vi "Write_Results_file.vi"(0 "Experiment start time":dbl, 1 "Experiment End time":dbl, 3 "Setup filename":string) -> ()   [LabVIEW 2016]
uses:
  Globals/Meas_global.vi
  Globals/Dynamic_call_global.ph.vi
  Controls/Post_Process.ctl
  Globals/Trav_pos_global.vi
  Controls/Inst_type.ctl
panel:
  out "x-y":u32
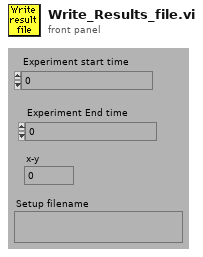
[diagram p1: front panel]
types:
  T1 = typedef "Post_Process.ctl" = enum16{"Take New Data", "Post Process Raw Data File"}
  T2 = enum16{"Save no data", "Save data in new files", "Save data in existing files"}
  T3 = typedef "Inst_type.ctl" = enum16{"Propeller anemometer", "Raw voltage", "Pressure Transducer", "Pitot-static tube", "Preston tube", "Hot wire", "Cross wire 1", "Cross wire 2", "Generic Linear", "Generic Polynomial", "Generic BackPoly", "Fast FID", "Thermocouple", "Cold wire", "Pulsed Wire", "LDA Vel", "LDA Tran time", "LDA Arr time", "Microphone"}
  T4 = typedef "Analysis_info_cluster.ctl" = cluster{"Colour":u32, "Inst type":T3, "Inst name":string, "Symbol":string, "Code name":string, "Extra Info":string, "Inst Array":T5, "Extra Titles":string[], "Extra Values":string[], "U":dbl, "u^2":dbl, "u^3":dbl, "u^4":dbl, "Skew_u":dbl, "Kurt_u":dbl, "Sd Error in Mean":dbl, "% u'/U":dbl, "X":dbl, "Y":dbl, "Z":dbl, "Timescale integral Estimate":dbl, "Sd Error in Variance":dbl, "Calib File":path, "Calib Constants":dbl[], "Output Position":bool, "Full Stats":bool, "Av Sampling Rate":dbl, "Av No of Samples":dbl, "Total Meas Time (s)":dbl, "ADAM Ch Name":string, "Max value":dbl, "Min value":dbl}
  T5 = typedef "Instrument_Array.ctl" = enum16{"PWA", "LDA", "Analogue"}
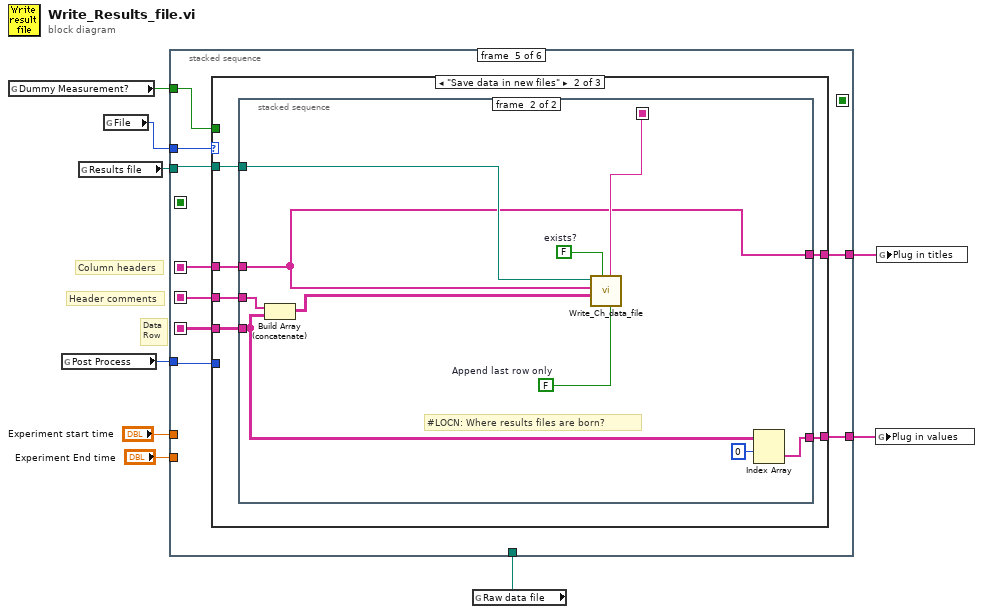
[diagram p0: block diagram]
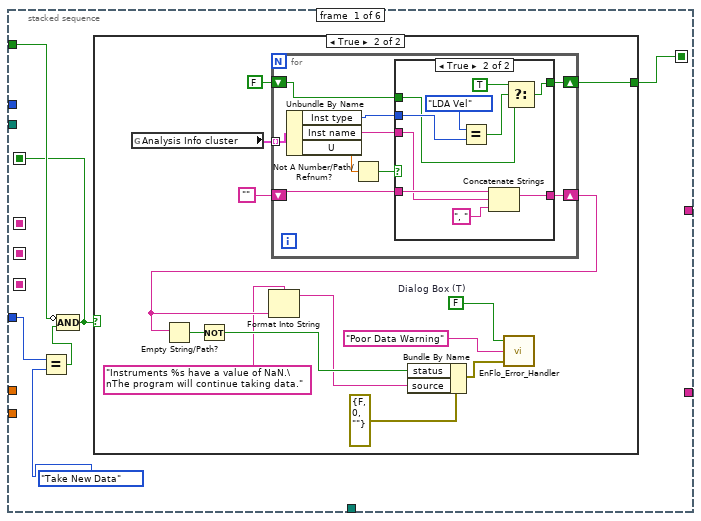
[diagram p2: hidden frame]
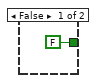
[diagram p3: hidden frame]
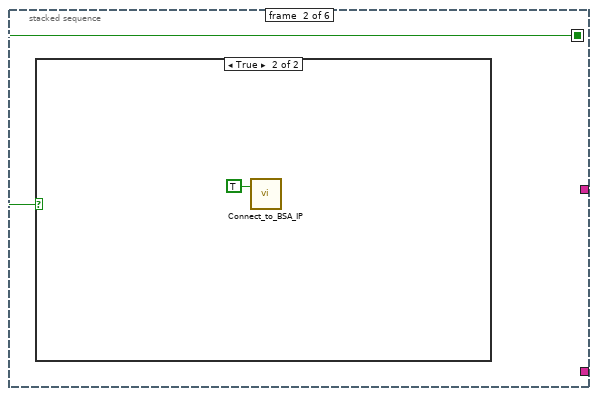
[diagram p5: hidden frame]
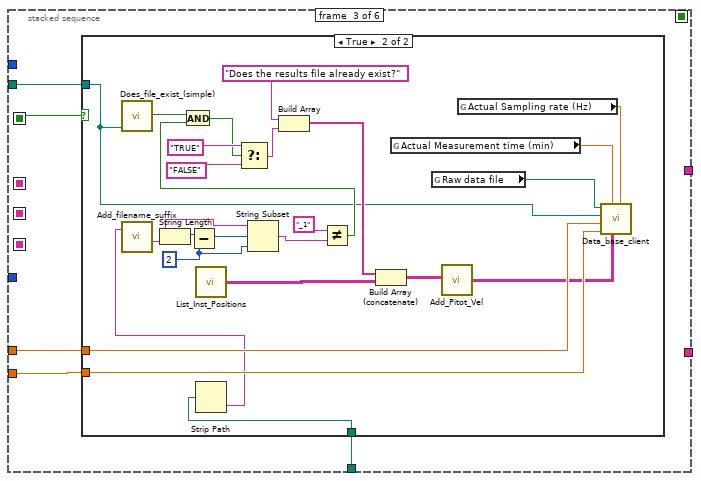
[diagram p7: hidden frame]
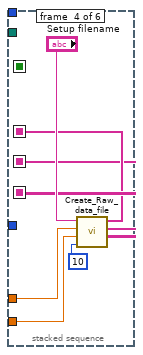
[diagram p9: hidden frame]
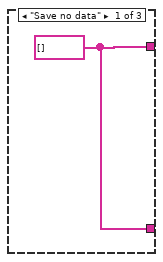
[diagram p10: hidden frame]
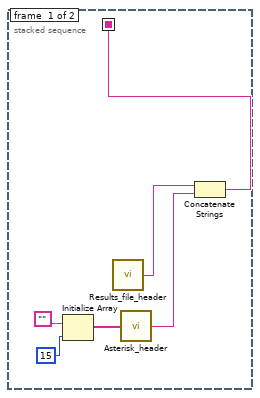
[diagram p11: hidden frame]
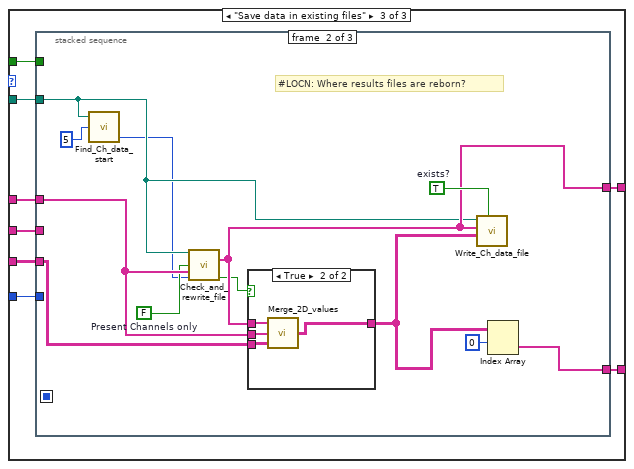
[diagram p12: hidden frame]
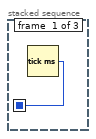
[diagram p13: hidden frame]
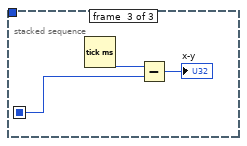
[diagram p15: hidden frame]
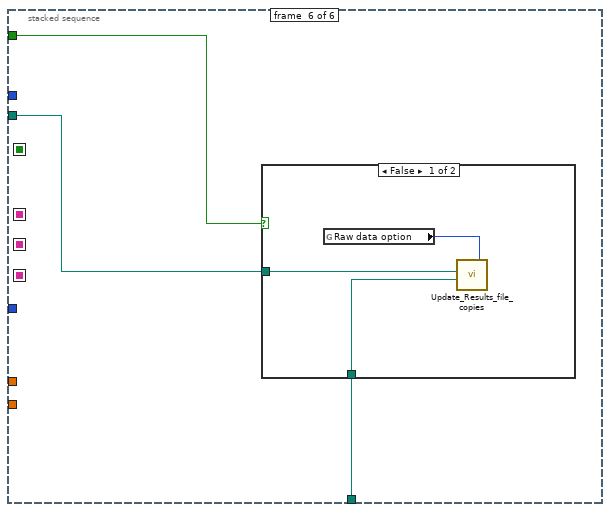
[diagram p16: hidden frame]
diagram:
  # "Data\nRow"
  # "Header comments"
  # "Column headers"
  n1 = global read "Trav_pos_global.vi" "Dummy Measurement?"() -> (w1:bool)
  n2 = global read "Meas_global.vi" "Post Process"() -> (w5:T1)
  n3 = global read "Meas_global.vi" "Results file"() -> (w2:path)
  n4 = global read "Meas_global.vi" "File"() -> (w9:T2)
  n5 = global read "Meas_global.vi" "Raw data file"() -> (w8:path)
  n6 = stacked-sequence {
    seq-local: [_ _ _ w84 _ _] -> [_ _ _ _ w97 _]
    seq-local: [_ _ _ w85 _ _] -> [_ _ _ _ w96 _]
    seq-local: [_ _ _ w83 _ _] -> [_ _ _ _ w95 _]
    seq-local: [w11 _ _ _ _ _] -> [_ _ w54 _ _ _]
    seq-local: [w10 _ _ _ _ _] -> [_ w51 _ _ _ _]
    tunnel: w9 -> [_ _ _ _ w98 _]
    tunnel: w8 -> [_ _ w53 _ _ w153]
    tunnel: "Experiment start time" -> [_ _ w57 w89 _ _]
    tunnel: "Experiment End time" -> [_ _ w56 w88 _ _]
    tunnel: w5 -> [w14 _ _ _ w94 _]
    tunnel: [_ _ _ _ w93 _] -> w4
    tunnel: [_ _ _ _ w92 _] -> w3
    tunnel: w2 -> [_ _ w55 _ w91 w152]
    tunnel: w1 -> [w12 _ _ _ w90 w151]
    frame #0 {
      n7 = Equal?(x=w14, y=Post_Process."Take New Data" ("Post Process")) -> (x = y?=w13:bool)
      n8 = Compound Arithmetic op=AND(invert w12, w13) -> (w11:bool)
      n9 = case shown="True" w11 {
        tunnel: [FALSE w17] -> w10
        frame False {
        }
        frame True {
          w26 = FALSE  # Dialog Box (T)
          n10 = global read "Meas_global.vi" "Analysis Info cluster"() -> (w29:T4[])
          n11 = for {
            tunnel: w29 -> [w38] mode=indexing
            shift-right: [w33] -> w21
            shift-left: "" -> [w35]
            shift-right: [w31] -> w17
            shift-left: FALSE -> [w30]
            n12 = Unbundle By Name(w38) -> ("Inst type"=w32:T3, "Inst name"=w34:string, "U"=w37:dbl)
            n13 = Not A Number/Path/Refnum?(number/path/refnum=w37) -> (NaN/Path/Refnum?=w36:bool)
            n14 = case shown="True" w36 {
              tunnel: w35 -> [w40 w50]
              tunnel: w34 -> [_ w49]
              tunnel: [w40 w47] -> w33
              tunnel: w32 -> [_ w45]
              tunnel: [w39 w42] -> w31
              tunnel: w30 -> [w39 w41]
              frame False {
              }
              frame True {
                n15 = Equal?(x=Inst_type."LDA Vel" ("Inst type"), y=w45) -> (x = y?=w44:bool)
                n16 = Concatenate Strings(w50, w49, ", " ("Substring")) -> (w47:string)
                n17 = Select(t=TRUE, s=w44, f=w41) -> (s? t:f=w42:bool)
              }
            }
          }
          n18 = Empty String/Path?(string/path=w21) -> (empty?=w23:bool)
          n19 = Not(x=w23) -> (.not. x?=w22:bool)
          n20 = Format Into String(format string="Instruments %s have a value of NaN.\nThe program will continue taking data." ("Format String"), w21) -> (resulting string=w19:string)  [unwired: 2 in, 1 out]
          n21 = Bundle By Name(cluster=errorcluster {"status"=FALSE, "code"=0, "source"=""} ("error in (no error)"), "status"=w22, "source"=w19) -> (w24:errorcluster)
          n22 = call "EnFlo_Error_Handler.vi"("error in (no error)"=w24, "Error Type"="Poor Data Warning", "Dialog Box (T)"=w26) -> ()  [unwired: 3 out]
        }
      }
    }
    frame #1 {
      n23 = case shown="True" w51 {
        frame False {
        }
        frame True {
          n24 = call "Connect_to_BSA_IP.vi"("Force Reconnect"=TRUE) -> ()  [unwired: 1 in, 2 out]
        }
      }
    }
    frame #2 {
      n25 = case shown="True" w54 {
        tunnel: w57 -> [_ w80]
        tunnel: w56 -> [_ w79]
        tunnel: w55 -> [_ w59]
        tunnel: w53 -> [_ w70]
        frame False {
        }
        frame True {
          w65 = 2 ("y")
          n26 = call "Does_file_exist_(simple).vi"("Pathname"=w59) -> ("exists?"=w62:bool)
          n27 = call "List_Inst_Positions.vi"() -> ("Position Info"=w74:string[][])  [unwired: 1 in]
          n28 = Strip Path(path=w70) -> (name=w69:string)  [unwired: 1 out]
          n29 = call "Add_filename_suffix.vi"("Filename"=w69) -> ("Base name"=w68:string)  [unwired: 1 in, 3 out]
          n30 = String Length(string=w68) -> (length=w67:i32)
          n31 = Subtract(x=w67, y=w65) -> (x-y=w66:i32)
          n32 = String Subset(string=w68, offset (0)=w66, length (rest)=w65) -> (substring=w64:string)
          n33 = Not Equal?(x="_1", y=w64) -> (x != y?=w61:bool)
          n34 = And(x=w62, y=w61) -> (x .and. y?=w60:bool)
          n35 = Select(t="TRUE", s=w60, f="FALSE") -> (s? t:f=w77:string)
          n36 = Build Array("Does the results file already exist?", w77) -> (w73:string[])
          n37 = Build Array (concatenate)(w73, w74) -> (w72:string[][])
          n38 = global read "Meas_global.vi" "Actual Measurement time (min)"() -> (w82:dbl)
          n39 = global read "Meas_global.vi" "Raw data file"() -> (w58:path)
          n40 = call "Add_Pitot_Vel.vi"("Channels from Client In"=w72) -> ("Channels from Client Out"=w71:string[][])
          n41 = global read "Meas_global.vi" "Actual Sampling rate (Hz)"() -> (w81:dbl)
          n42 = call "Data_base_client.vi"("Average Sampling freq"=w81, "Channels from Client"=w71, "Average Meas Time (min)"=w82, "End time"=w79, "Start time"=w80, "Results File Pathname"=w59, "Raw Data Pathname"=w58) -> ()  [unwired: 4 out]
        }
      }
    }
    frame #3 {
      n43 = call "Create_Raw_data_file.vi"("No of averages"=10, "End time"=w88, "Start time"=w89, "Setup filename"="Setup filename") -> ("Values"=w85:string[][], "Header Comments"=w83:string[], "Column headers"=w84:string[])  [unwired: 1 out]
    }
    frame #4 {
      n44 = case shown="\"Save data in new files\"" w98 {
        tunnel: w97 -> [_ w105 w129]
        tunnel: w96 -> [_ w104 w128]
        tunnel: w95 -> [_ w103 w127]
        tunnel: w91 -> [_ w102 w126]
        tunnel: w94 -> [_ _ w125]
        tunnel: [w99 w100 w124] -> w93
        tunnel: [w99 w101 w123] -> w92
        tunnel: w90 -> [_ _ w122]
        frame "Save no data" {
          w99 = string[] [] ("Merged Channels")
        }
        frame "Save data in new files" {
          n45 = stacked-sequence {
            seq-local: [w106 _] -> [_ w118]
            tunnel: w105 -> [_ w115]
            tunnel: w104 -> [_ w113]
            tunnel: w103 -> [_ w120]
            tunnel: w102 -> [_ w116]
            tunnel: [_ w115] -> w101
            tunnel: [_ w112] -> w100
            frame #0 {
              n46 = Initialize Array("", 15) -> (w110:string[])
              n47 = call "Results_file_header.vi"() -> ("Header"=w111:string)
              n48 = call "Asterisk_header.vi"("Channel names"=w110) -> ("Header string"=w107:string)
              n49 = Concatenate Strings(w111, w107) -> (w106:string)
            }
            frame #1 {
              w117 = FALSE  # Append last row only
              w121 = FALSE  # exists?
              # "#LOCN: Where results files are born?"
              n50 = Build Array (concatenate)(w120, w113) -> (w119:string[][])
              n51 = call "Write_Ch_data_file.vi"("Append last row only"=w117, "Header string"=w118, "exists?"=w121, "Channel Values"=w119, "Channel names"=w115, "Filename"=w116) -> ()  [unwired: 2 in, 4 out]
              n52 = Index Array(array=w113, index (row)=0) -> (element=w112:string[])  [unwired: 1 in]
            }
          }
        }
        frame "Save data in existing files" {
          n53 = stacked-sequence {
            seq-local: [w130 _ _] -> [_ _ w149]
            tunnel: w129 -> [_ w140 _]
            tunnel: w128 -> [_ w141 _]
            tunnel: w127 -> [_ _ _]
            tunnel: w126 -> [_ w137 _]
            tunnel: w125 -> [_ _ _]
            tunnel: [_ w131 _] -> w124
            tunnel: [_ w139 _] -> w123
            tunnel: w122 -> [_ _ _]
            frame #0 {
              n54 = Tick Count (ms)() -> (millisecond timer value=w130:u32)
            }
            frame #1 {
              w138 = FALSE  # Present Channels only
              w142 = TRUE  # exists?
              # "#LOCN: Where results files are reborn?"
              n55 = call "Find_Ch_data_start.vi"("Approx No Of Columns"=5, "Filename"=w137) -> ("Start of read offset output"=w135:i32)  [unwired: 1 in, 2 out]
              n56 = call "Check_and_rewrite_file.vi"("Filename"=w137, "Present Channels only"=w138, "Present Channels"=w140, "Start of read offset (chars.: 0)"=w135) -> ("Merged Channels"=w139:string[], "Merged?"=w134:bool)  [unwired: 10 out]
              n57 = case shown="True" w134 {
                tunnel: w141 -> [w143 w145]
                tunnel: w140 -> [_ w146]
                tunnel: [w143 w144] -> w132
                tunnel: w139 -> [_ w147]
                frame False {
                }
                frame True {
                  n58 = call "Merge_2D_values.vi"("Values In"=w145, "Present Channels"=w146, "Desired Channels"=w147) -> ("Values Out"=w144:string[][])
                }
              }
              n59 = call "Write_Ch_data_file.vi"("exists?"=w142, "Channel Values"=w132, "Channel names"=w139, "Filename"=w137) -> ()  [unwired: 4 in, 4 out]
              n60 = Index Array(array=w132, index (row)=0) -> (element=w131:string[])  [unwired: 1 in]
            }
            frame #2 {
              n61 = Tick Count (ms)() -> (millisecond timer value=w150:u32)
              n62 = Subtract(x=w150, y=w149) -> (x-y=→"x-y":u32)
            }
          }
        }
      }
    }
    frame #5 {
      n63 = case shown="False" w151 {
        tunnel: w153 -> [w156 _]
        tunnel: w152 -> [w154 _]
        frame False {
          n64 = global read "Meas_global.vi" "Raw data option"() -> (w155:enum16{"Save raw data", "Raw data not saved"})
          n65 = call "Update_Results_file_copies.vi"("Raw data option"=w155, "Raw data file"=w156, "Results file"=w154) -> ()  [unwired: 4 out]
        }
        frame True {
        }
      }
    }
  }
  n66 = global write "Dynamic_call_global.ph.vi" "Plug in values"(w4) -> ()
  n67 = global write "Dynamic_call_global.ph.vi" "Plug in titles"(w3) -> ()
